vi "Get I32 Notifier Ref.vi"(8 "error in (no error)":errorcluster, 9 "element data type":i32, 10 "Tag Name":string, 11 "Current Value Table in":refnum<class "Current Value Table.lvclass">) -> (0 "error out":errorcluster, 2 "notifier out":refnum<notifier>, 3 "Current Value Table out":refnum<class "Current Value Table.lvclass">)   [LabVIEW 2024, in "Current Value Table.lvlib" / "Current Value Table.lvclass"]
uses:
  Current Value Table.lvclass
  CVT_I32/CVT_I32.lvclass
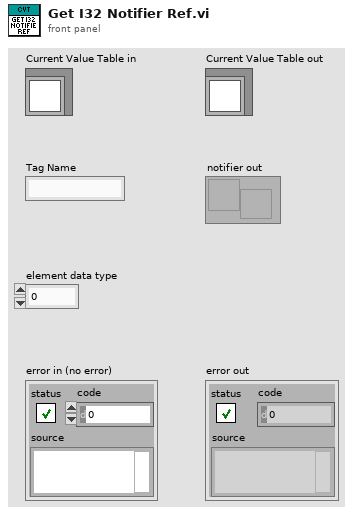
[diagram p1: front panel]
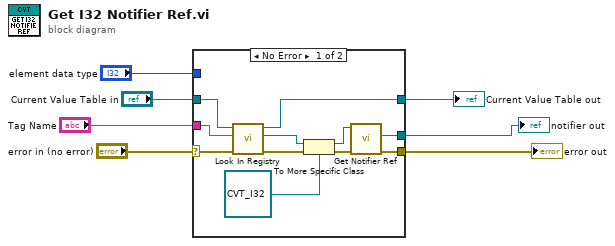
[diagram p0: block diagram]
diagram:
  n1 = case shown="No Error" "error in (no error)" {
    selector: "error in (no error)" -> [w9 w20]
    tunnel: [w8 w20] -> w6
    tunnel: [w13 w19] -> w4
    tunnel: "Current Value Table in" -> [w17 w19]
    tunnel: "Tag Name" -> [w16 _]
    tunnel: [w10 _] -> w2
    tunnel: "element data type" -> [_ _]
    frame No Error {
      n2 = call-dynamic "Look In Registry.vi"("error in (no error)"=w9, "Tag Name"=w16, "Current Value Table in"=w17) -> ("error out"=w14:errorcluster, "CVT_Item out"=w15:refnum<class "iCVT_Item.lvclass">, "Current Value Table out"=w13:refnum<class "Current Value Table.lvclass">)  [unwired: 5 in, 1 out]
      n3 = To More Specific Class(target class=refnum<class "CVT_I32.lvclass"> refnum ("Current Value Table.lvlib:CVT_I32.lvclass"), reference=w15, error in=w14) -> (specific class reference=w11:refnum<class "CVT_I32.lvclass">, error out=w12:errorcluster)
      n4 = call-dynamic "Get Notifier Ref.vi"("error in (no error)"=w12, "CVT_I32 in"=w11) -> ("error out"=w8:errorcluster, "notifier out"=w10:refnum<notifier>)  [unwired: 7 in, 1 out]
    }
    frame Error {
    }
  }
  "error out" <- w6
  "Current Value Table out" <- w4
  "notifier out" <- w2
